vi "test_ServiceLocationPool_GetLocationTwice_ReturnsCachedLocation.vi"(8 "error in (no error)":errorcluster) -> (0 "error out":errorcluster, 2 "result":string, 3 "pass":bool)   [LabVIEW 2020, in "MeasurementServerTests.lvlib"]
uses:
  MeasurementServerTests.lvlib
  Runtime/MeasurementLink Discovery/MeasurementLink Discovery.lvlib
  Runtime/MeasurementLink Discovery Client/RPC Messages/ni_measurementlink_discovery_v1_ResolveServiceRequest.ctl
  Runtime/MeasurementLink Discovery Client/MeasurementLink Discovery Client.lvlib
  Runtime/MeasurementLink Measurement Server/MeasurementLink Measurement Server.lvlib
  Runtime/MeasurementLink Discovery/Service Location FGV Action.ctl
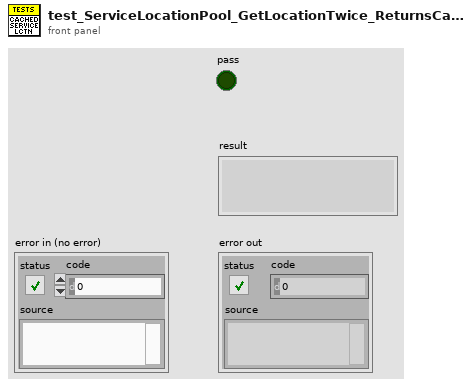
[diagram p1: front panel]
types:
  T1 = typedef "MeasurementLink Discovery Client.lvlib/ni_measurementlink_discovery_v1_ResolveServiceRequest.ctl" = cluster{"provided_interface":string, "service_class":string}
  T2 = typedef "MeasurementLink Discovery.lvlib/Service Location FGV Action.ctl" = enum16{"Get Service Location", "Reresolve Service Location"}
  T3 = typedef "MeasurementLink Discovery Client.lvlib/ni_measurementlink_discovery_v1_ServiceLocation.ctl" = cluster{"location":string, "insecure_port":string, "ssl_authenticated_port":string}
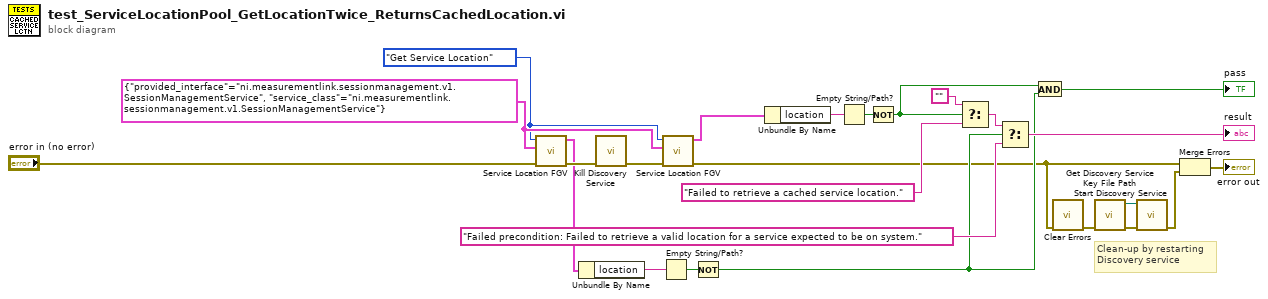
[diagram p0: block diagram]
diagram:
  w17 = T1 {"provided_interface"="ni.measurementlink.sessionmanagement.v1.SessionManagementService", "service_class"="ni.measurementlink.sessionmanagement.v1.SessionManagementService"} ("Resolve Service Request")
  w16 = Service_Location_FGV_Action."Get Service Location" ("Action")
  # "Clean-up by restarting\nDiscovery service"
  n1 = call "Service Location FGV.vi"("error in"="error in (no error)", "resolve service request"=w17, "action"=w16) -> ("error out"=w20:errorcluster, "service location"=w13:T3)  [unwired: 6 in, 1 out]
  n2 = Unbundle By Name(w13) -> ("location"=w14:string)
  n3 = call "Kill Discovery Service.vi"("error in"=w20) -> ("error out"=w19:errorcluster)  [unwired: 10 in]
  n4 = Empty String/Path?(string/path=w14) -> (empty?=w15:bool)
  n5 = call "Service Location FGV.vi"("error in"=w19, "resolve service request"=w17, "action"=w16) -> ("error out"=w1:errorcluster, "service location"=w18:T3)  [unwired: 6 in, 1 out]
  n6 = Not(x=w15) -> (.not. x?=w7:bool)
  n7 = Unbundle By Name(w18) -> ("location"=w24:string)
  n8 = Empty String/Path?(string/path=w24) -> (empty?=w23:bool)
  n9 = Not(x=w23) -> (.not. x?=w8:bool)
  n10 = Select(t="", s=w8, f="Failed to retrieve a cached service location.") -> (s? t:f=w12:string)
  n11 = Select(t=w12, s=w7, f="Failed precondition: Failed to retrieve a valid location for a service expected to be on system.") -> (s? t:f=→"result":string)
  n12 = And(x=w8, y=w7) -> (x .and. y?=→"pass":bool)
  n13 = call <vilib>:"Clear Errors.vi"("error in (no error)"=w1) -> ("error out"=w2:errorcluster)  [unwired: 5 in, 1 out]
  n14 = call "Get Discovery Service Key File Path.vi"("error in (no error)"=w2) -> ("error out"=w6:errorcluster, "key file path"=w5:path)  [unwired: 9 in]
  n15 = call "Start Discovery Service.vi"("error in"=w6, "key file path"=w5) -> ("error out"=w3:errorcluster)  [unwired: 9 in]
  n16 = Merge Errors(w1, w3) -> (→"error out":errorcluster)
